vi "teardown.vi"(8 "error in (no error)":errorcluster, 11 "VISA resource name":refnum<visa-resource-name>) -> ()   [LabVIEW 2019, in "SpectraPro.lvlib"]
uses:
  SpectraPro.lvlib
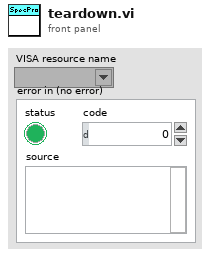
[diagram p1: front panel]
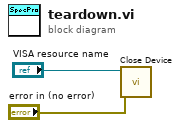
[diagram p0: block diagram]
diagram:
  n1 = call "Close Device.vi"("error in (no error)"="error in (no error)", "VISA resource name"="VISA resource name") -> ()  [unwired: 10 in]
